vi "Version Text.vi"(6 "LabPack Shared Library":path=path "", 8 "Error In":errorcluster) -> (0 "Error Out":errorcluster, 3 "Version":string)   [LabVIEW 2019, in "LabPack.lvlib"]
doc: "Gets the version number of the LabPack shared library as a string in dot notation, i.e. \"Major.Minor.Patch\". The LabPack shared library maintains a semantic versioning number with a Major, Minor, and Patch component. A difference in the Major number indicates backwards compatible breaking changes. A difference in the Minor number indicates new features and fixes that do not break backwards compatibility. A difference in the Patch number indicates a fix that does not break backwards compatibility and does not add any new features."
uses:
  LabPack.lvlib
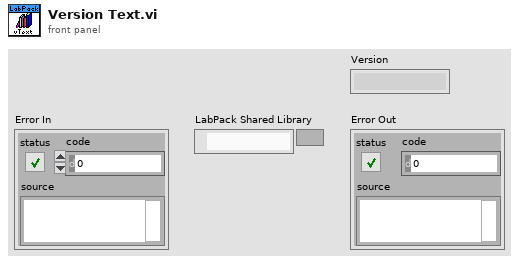
[diagram p1: front panel]
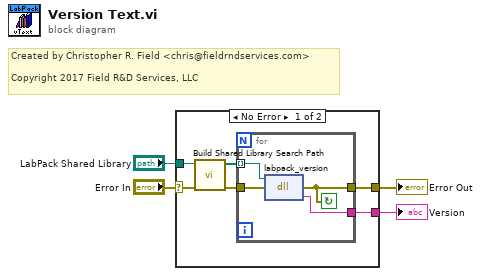
[diagram p0: block diagram]
diagram:
  # "Created by Christopher R. Field <chris@fieldrndservices.com>\n\nCopyright 2017 Field R&D Services, LLC"
  n1 = case shown="No Error" "Error In" {
    selector: "Error In" -> [w9 w15]
    tunnel: "LabPack Shared Library" -> [w10 _]
    tunnel: [w6 w15] -> w2
    tunnel: [w5 _] -> w1
    frame No Error {
      n2 = call "Build Shared Library Search Path.vi"("Error In"=w9, "LabPack Shared Library"=w10) -> ("Error Out"=w8:errorcluster, "Search Path"=w7:path[])  [unwired: 8 in]
      n3 = for {
        tunnel: w8 -> [w14]
        tunnel: w7 -> [w13] mode=indexing
        tunnel: [w12] -> w6
        tunnel: [w11] -> w5
        stop <- w12 continue-if-true
        n4 = dll-call lib="D:/Users/cfield/Code/MessagePack/LabPack/LabVIEW/trunk/src/LabPack/Private/labpack-x64.dll" fn="labpack_version"(path in=w13, error in=w14) -> (error out=w12:errorcluster, "return type"=w11:string)  [unwired: 1 in, 1 out]
      }
    }
    frame Error {
    }
  }
  "Error Out" <- w2
  "Version" <- w1
